vi "Self Configure.vi"(8 "error in":errorcluster, 11 "AnalogInput in":refnum<class "AnalogInput.lvclass">) -> (0 "error out":errorcluster, 3 "AnalogInput out":refnum<class "AnalogInput.lvclass">)   [LabVIEW 2019, in "AnalogInput.lvlib" / "AnalogInput.lvclass"]
uses:
  Library/AnalogInput.lvclass
  C:/Users/Public/Documents/Development/builds/Instruments/Instruments.lvlibp/Library/Instruments.lvclass
  Custom Controls/Configuration Keys.ctl
  Library/AnalogInput.lvclass/AnalogInput.ctl
  builds/Instruments/Instruments.lvlibp/Accessors/Write Padding_enable.vi
  builds/Instruments/Instruments.lvlibp/Private/Accessors/Read Poll(ms).vi
  builds/Instruments/Instruments.lvlibp/Library/Instruments.lvclass
  builds/Tools/Config.lvlibp/Config.lvclass
  C:/Users/Public/Documents/Development/builds/Tools/Config.lvlibp/Config.lvclass
panel:
  in  "Configuration Keys":T1
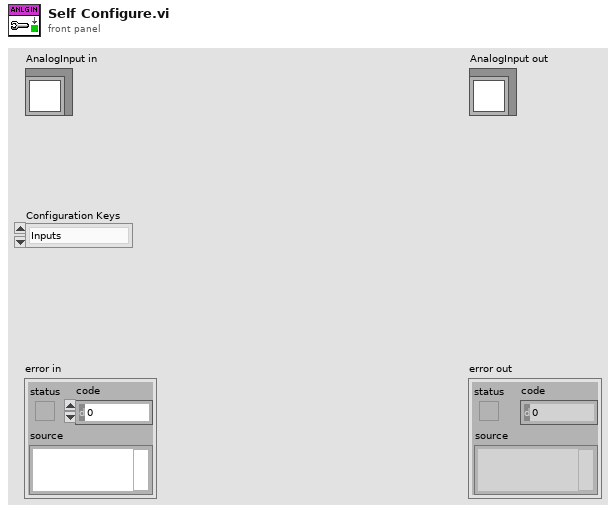
[diagram p1: front panel]
types:
  T1 = typedef "AnalogInput.lvlib/AnalogInput.lvclass/Configuration Keys.ctl" = enum16{"Inputs", "Filter", "Rate", "DigitalTriggerEn"}
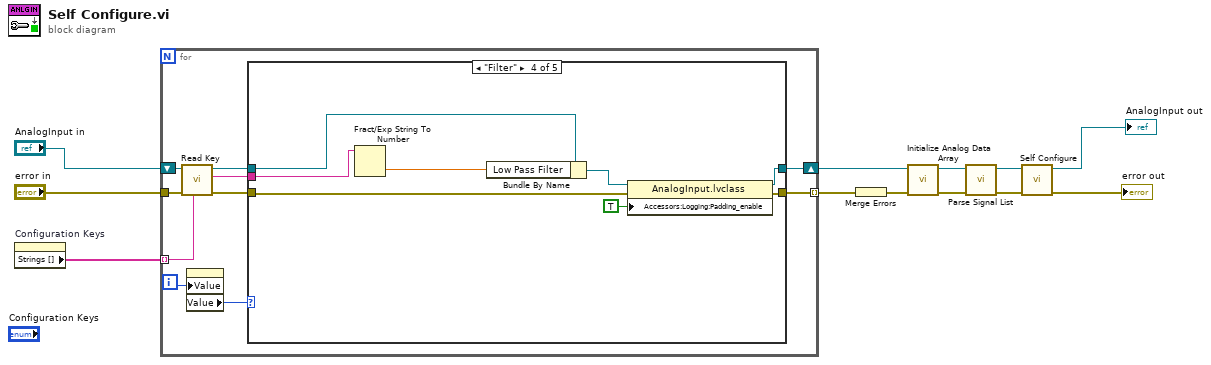
[diagram p0: block diagram]
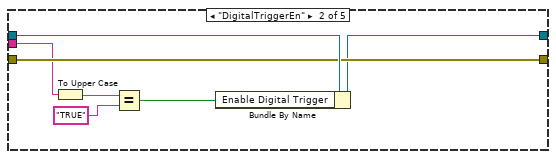
[diagram p3: hidden frame]
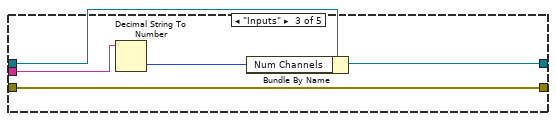
[diagram p4: hidden frame]
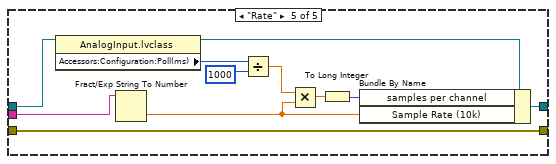
[diagram p5: hidden frame]
diagram:
  n1 = property on="Configuration Keys" class="Enum (strict)"() -> ("Strings []"=w10:string[])  [unwired: 2 in, 2 out]
  n2 = for {
    tunnel: w10 -> [w18] mode=indexing
    tunnel: "error in" -> [w21]
    shift-right: [w17] -> w7
    shift-left: "AnalogInput in" -> [w22]
    tunnel: [w16] -> w6 mode=indexing
    i -> [w14]
    n3 = call "Read Key.vi"("Key Name"=w18, "error in"=w21, "Config in"=w22) -> ("error out"=w19:errorcluster, "Key Value"=w15:string, "Config out"=w20:refnum<class "AnalogInput.lvclass">)  [unwired: 6 in]
    n4 = property on="Configuration Keys" class="Enum (strict)"("Value"=w14) -> ("Value"=w13:T1)  [unwired: 2 in, 2 out]
    n5 = case shown="\"Filter\"" w13 {
      tunnel: w20 -> [w24 w31 w35 w44 w52]
      tunnel: w19 -> [w23 w30 w36 w39 w55]
      tunnel: [w24 w26 w34 w40 w54] -> w17
      tunnel: [w23 w30 w36 w38 w55] -> w16
      tunnel: w15 -> [_ w29 w33 w43 w53]
      frame Default {
      }
      frame "DigitalTriggerEn" {
        n6 = To Upper Case(1:w29) -> (0:w28:string)
        n7 = Equal?(x=w28, y="TRUE") -> (x = y?=w25:bool)
        n8 = Bundle By Name(cluster=w31, "Enable Digital Trigger"=w25) -> (w26:refnum<class "AnalogInput.lvclass">)
      }
      frame "Inputs" {
        n9 = Decimal String To Number(string=w33) -> (number=w32:i32)  [unwired: 2 in, 1 out]
        n10 = Bundle By Name(cluster=w35, "Num Channels"=w32) -> (w34:refnum<class "AnalogInput.lvclass">)
      }
      frame "Filter" {
        n11 = Fract/Exp String To Number(string=w43) -> (number=w42:dbl)  [unwired: 3 in, 1 out]
        n12 = Bundle By Name(cluster=w44, "Low Pass Filter"=w42) -> (w41:refnum<class "AnalogInput.lvclass">)
        n13 = property class="AnalogInput.lvclass"(reference=w41, error in=w39, "Accessors:Logging:Padding_enable"=TRUE ("Instrument:Logging:Padding:Enable")) -> (reference out=w40:refnum<class "AnalogInput.lvclass">, error out=w38:errorcluster)
      }
      frame "Rate" {
        n14 = property class="AnalogInput.lvclass"(reference=w52) -> (reference out=w51:refnum<class "AnalogInput.lvclass">, "Accessors:Configuration:Poll(ms)"=w50:u32)  [unwired: 1 in, 1 out]
        n15 = Fract/Exp String To Number(string=w53) -> (number=w47:dbl)  [unwired: 3 in, 1 out]
        n16 = Divide(x=w50, y=u32 1000) -> (x/y=w48:dbl)
        n17 = Multiply(x=w48, y=w47) -> (x*y=w45:dbl)
        n18 = To Long Integer(number=w45) -> (32bit integer=w46:i32)
        n19 = Bundle By Name(cluster=w51, "samples per channel"=w46, "Sample Rate (10k)"=w47) -> (w54:refnum<class "AnalogInput.lvclass">)
      }
    }
  }
  n20 = Merge Errors(w6) -> (w5:errorcluster)
  n21 = call "Initialize Analog Data Array.vi"("error in"=w5, "AnalogInput in"=w7) -> ("error out"=w3:errorcluster, "AnalogInput out"=w4:refnum<class "AnalogInput.lvclass">)  [unwired: 8 in]
  n22 = call "Parse Signal List.vi"("error in"=w3, "AnalogInput in"=w4) -> ("error out"=w1:errorcluster, "AnalogInput out"=w2:refnum<class "AnalogInput.lvclass">)  [unwired: 8 in]
  n23 = call-parent "Self Configure.vi"("error in"=w1, "Instruments in"=w2) -> ("error out"=→"error out":errorcluster, "Instruments out"=→"AnalogInput out":refnum<class "AnalogInput.lvclass">)  [unwired: 8 in]
